vi "saveNewTSR.vi"(0 "reference in":refnum<class "excelFile.lvclass">, 2 "TSR_details":T1={"Company/Institution:"="", "Address:"="", "Department:"="", "City:"="", "Post Code:"="", "Country:"="", "Contact:"="", "Ref:"="", "Issue description:"="", "Actions:"="", "TYPE:"="Repair", "Shipping:"=0, "Discount:"=0, "dataIN"=[], "Device type:"="microQuark", "Serial Number:"="", "PMC number:"="", "Labour Hours:"=0.0, "Service Location:"=FALSE, "start_hour"="", "end_hour"="", "o2_exp_date"="", "GST"=TRUE}, 5 "error in (no error)":errorcluster) -> (14 "reference out":refnum<class "excelFile.lvclass">, 16 "latest_TSR_path":string, 19 "error out":errorcluster)   [LabVIEW 2016, in "excelFile.lvclass"]
uses:
  excelFile.lvclass
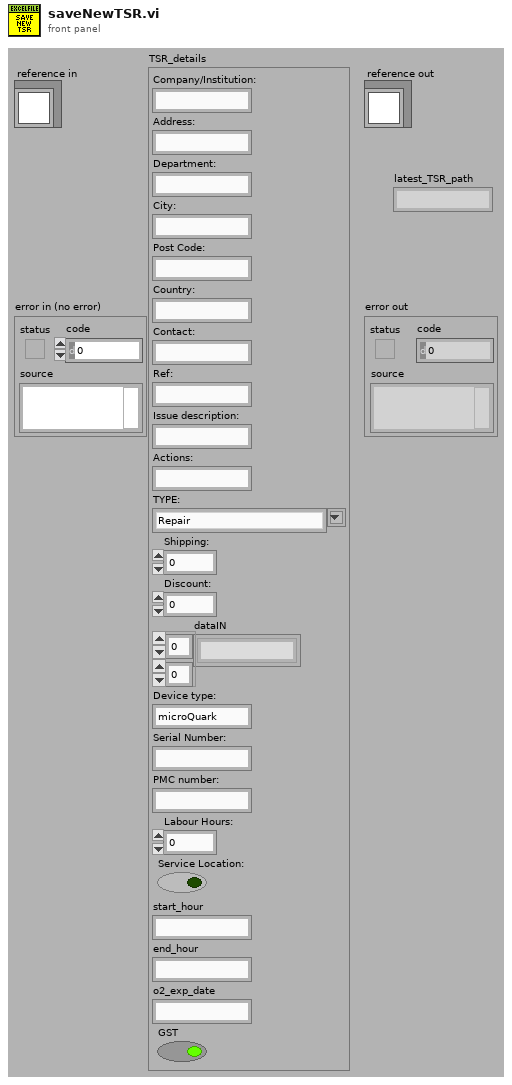
[diagram p1: front panel]
types:
  T1 = cluster{"Company/Institution:":string, "Address:":string, "Department:":string, "City:":string, "Post Code:":string, "Country:":string, "Contact:":string, "Ref:":string, "Issue description:":string, "Actions:":string, "TYPE:":string, "Shipping:":i32, "Discount:":i32, "dataIN":string[][], "Device type:":string, "Serial Number:":string, "PMC number:":string, "Labour Hours:":dbl, "Service Location:":bool, "start_hour":string, "end_hour":string, "o2_exp_date":string, "GST":bool}
  T2 = typedef "excelFile.lvclass/ObjectAttributesRef.ctl" = refnum<data-value>
  T3 = typedef "excelFile.lvclass/ObjectAttributes.ctl" = cluster{"MyAttribute":dbl, "path":string, "Refnum Excel":cluster{"Excel._Application":refnum<k7>, "Workbooks":refnum<k7>, "Open":refnum<k7>}, "data":string[][][], "save":bool, "fileType":T4, "rowsColor":u32[], "python_ref":refnum<class "python.lvclass">, "items_rows":i32[], "excel_range":i32[][], "TSR":cluster{"number":string, "TSR_path":path, "service_path":path, "email_to":string}, "excel_already_opened?":bool, "file_already_opened?":bool, "excel_protected_opened?":bool, "Refnum Cluster Worksheets":cluster{"Excel._Application":refnum<k7>, "Workbooks":refnum<k7>, "Open":refnum<k7>, "Worksheets":refnum<k7>, "Excel._Worksheet":refnum<k7>}, "#_rows_defective":i32, "#_rows_spare":i32}
  T4 = typedef "excelFile.lvclass/fileType.ctl" = enum16{"devices", "items", "partsTracking", "TSR"}
  T5 = cluster{"Excel._Application":refnum<k7>, "Workbooks":refnum<k7>, "Open":refnum<k7>, "Worksheets":refnum<k7>, "Excel._Worksheet":refnum<k7>}
  T6 = cluster{"number":string, "TSR_path":path, "service_path":path, "email_to":string}
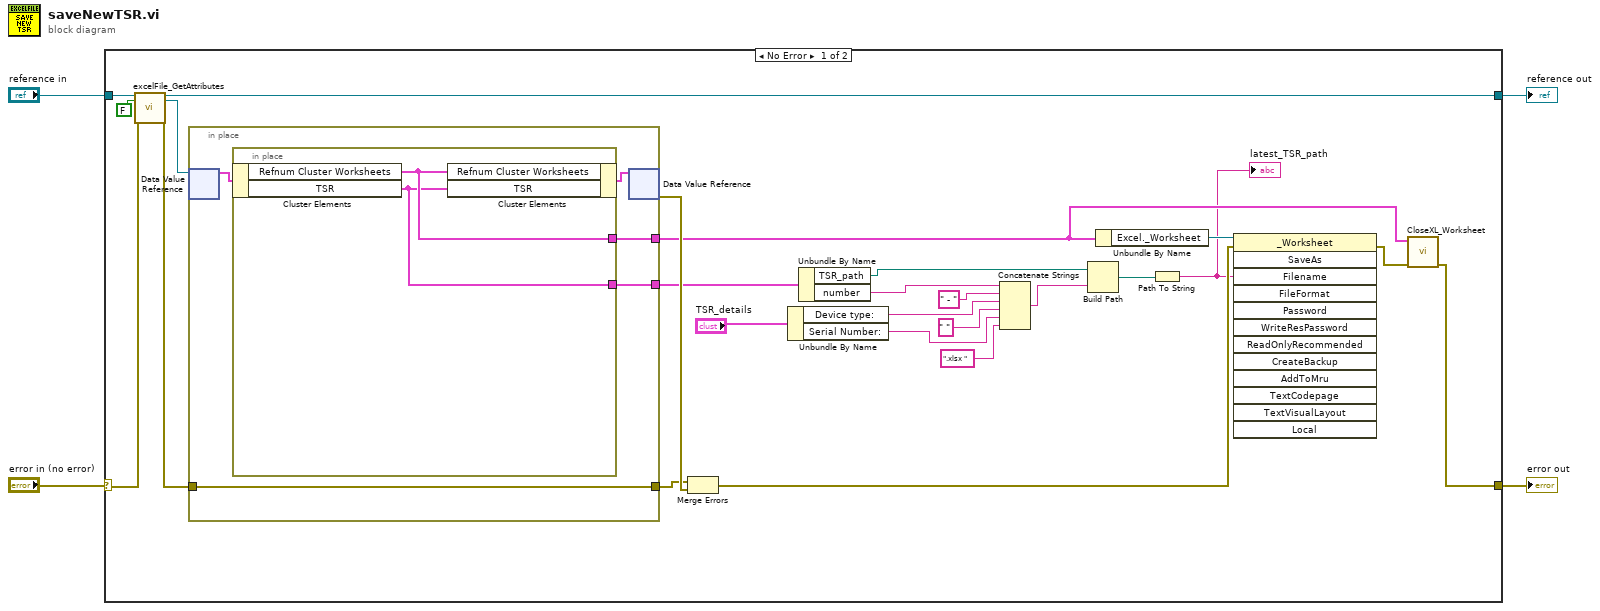
[diagram p0: block diagram]
diagram:
  n1 = case shown="No Error" "error in (no error)" {
    selector: "error in (no error)" -> [w25 w38]
    tunnel: [w7 w38] -> w3
    tunnel: [w23 w37] -> w1
    tunnel: "reference in" -> [w27 w37]
    frame No Error {
      n2 = call "excelFile_GetAttributes.vi"("reference in"=w27, "return data? (T)"=FALSE, "error in (no error)"=w25) -> ("reference out"=w23:refnum<class "excelFile.lvclass">, "attributes ref"=w22:T2, "error out"=w24:errorcluster)  [unwired: 13 in, 1 out]
      n3 = in-place {
        in-place-border: w24 -> [w32]
        in-place-border: [w32] -> w28
        in-place-border: [w31] -> w9
        in-place-border: [w30] -> w12
        n4 = in-place-dvr #1(w22) -> (w33:T3)  [unwired: 1 out]
        n5 = in-place {
          in-place-border: [w36] -> w31
          in-place-border: [w35] -> w30
          n6 = in-place-cluster #2(w33) -> ("Refnum Cluster Worksheets"=w36:T5, "TSR"=w35:T6)
          n7 = in-place-cluster #2("Refnum Cluster Worksheets"=w36, "TSR"=w35) -> (w34:T3)
        }
        n8 = in-place-dvr #1(w34) -> (w29:errorcluster)  [unwired: 1 out]
      }
      n9 = Merge Errors(w28, w29) -> (w8:errorcluster)
      n10 = Unbundle By Name("TSR_details") -> ("Device type:"=w18:string, "Serial Number:"=w16:string)
      n11 = Unbundle By Name(w12) -> ("TSR_path"=w11:path, "number"=w10:string)
      n12 = Concatenate Strings(w10, " - ", w18, " ", w16, ".xlsx ") -> (w14:string)
      n13 = Build Path(base path=w11, name or relative path=w14) -> (appended path=w13:path)
      n14 = Unbundle By Name(w9) -> ("Excel._Worksheet"=w21:refnum<k7>)
      n15 = Path To String(path=w13) -> (string=w6:string)
      "latest_TSR_path" <- w6
      n16 = invoke class="_Worksheet" method="SaveAs"(reference=w21, error in=w8, "Filename"=w6) -> (error out=w20:errorcluster)  [unwired: 10 in, 12 out]
      n17 = call <userlib>:"CloseXL_Worksheet.vi"("error in (no error)"=w20, "Refnum Cluster In"=w9) -> ("error out"=w7:errorcluster)  [unwired: 8 in, 1 out]
    }
    frame Error {
    }
  }
  "error out" <- w3
  "reference out" <- w1
